vi "PointerPosition.vi"(10 "Reframed Position (m)":cluster{"x (m)":dbl, "y (m)":dbl, "z (m)":dbl} {"z (m)" format="%.1p"; "y (m)" format="%.1p"; "x (m)" format="%.1p"}) -> (1 "y string":string, 2 "x string":string)   [LabVIEW 2021]
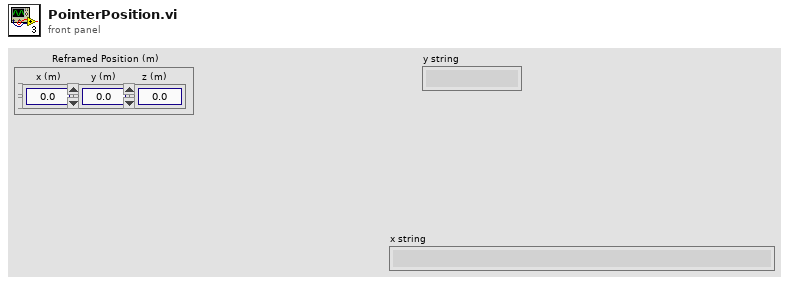
[diagram p1: front panel]
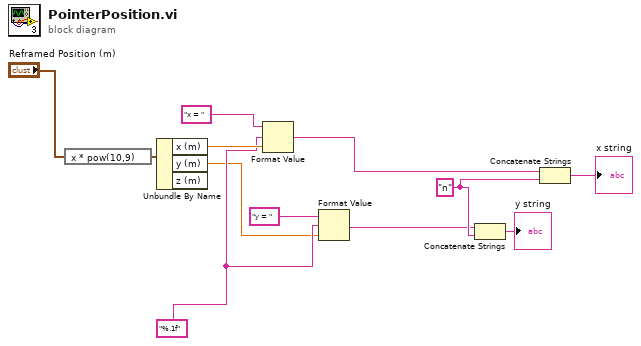
[diagram p0: block diagram]
diagram:
  w3 = "n" ("string")
  w5 = "%.1f" ("format string")
  n1 = expression code="x * pow(10,9)"("Reframed Position (m)") -> (w9:cluster{"x (m)":dbl, "y (m)":dbl, "z (m)":dbl})
  n2 = Unbundle By Name(w9) -> ("x (m)"=w11:dbl, "y (m)"=w4:dbl)  [unwired: 1 out]
  n3 = Format Value(string ("")="x = " ("string"), format string=w5, value (0)=w11) -> (output string=w8:string)
  n4 = Format Value(string ("")="y = " ("string"), format string=w5, value (0)=w4) -> (output string=w2:string)
  n5 = Concatenate Strings(w2, w3) -> (→"y string":string)
  n6 = Concatenate Strings(w8, w3) -> (→"x string":string)
